vi "Test Read Arrays.vi"(11 "TwinCAT ADS in":refnum<class "TwinCAT ADS.lvclass">) -> (3 "TwinCAT ADS out":refnum<class "TwinCAT ADS.lvclass">)   [LabVIEW 2018]
uses:
  TwinCAT ADS Class/TwinCAT ADS.lvclass
  Controls/ST_Complex.ctl
  Controls/Enum.ctl
  Controls/ST_Simple.ctl
  Controls/ST_Packed.ctl
  Controls/FB_Simple.ctl
  Controls/FB_Complex.ctl
  Controls/FB_Packed.ctl
  efa47bad-600a-438a-a84b-18a2d0bd5ed2.vi
  ee10bb5d-8528-4d89-b762-575e451c5044.vi
  55aabb0d-44ac-4cb0-b0b9-4848951ad384.vi
  322127f1-f009-44a9-8110-edacd942befb.vi
  88bbdbaa-0963-4497-b00e-77a7b5e38a5d.vi
  93c90ac2-55b6-4b22-b505-e684b3e479fa.vi
  1b7d90d0-fd5f-4b83-bacb-e5e8491709de.vi
  0e82c4fa-873b-4361-ac99-2e6e4b7cd392.vi
  da0f88be-82f8-4e5b-86e7-5baa69d9b51e.vi
  4782b519-43e7-4b8e-bd72-e209be860882.vi
  e7a7b24b-aede-49d7-b369-bb451e1de87e.vi
  TwinCAT ADS Class/VIs/Data/Read.vi
  <vilib>/addons/_JKI Toolkits/Caraya/classes/Assert/Assert Equal Value and Type_Variant.vi
  <vilib>/addons/_JKI Toolkits/Caraya/classes/Assert/Assert True.vi
  <vilib>/addons/_JKI Toolkits/Caraya/classes/Assert/Assert.lvclass
  <vilib>/addons/_JKI Toolkits/Caraya/classes/Test/Test.lvclass
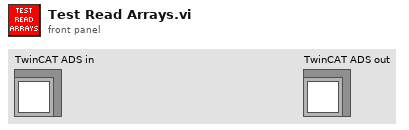
[diagram p1: front panel]
types:
  T1 = typedef "FB_Complex.ctl" = cluster{"_fMember":dbl, "_stMember":T2, "_fbSimpleMember":T6, "_fbPackedMember":T7}
  T2 = typedef "ST_Complex.ctl" = cluster{"bMember":bool, "eMember":T3, "stSimpleMember":T4, "stPackedMember":T5, "FB_Simple":T6, "arrfMember":dbl[]}
  T3 = typedef "Enum.ctl" = enum16{"Member 0", "Member 1", "Member 2"}
  T4 = typedef "ST_Simple.ctl" = cluster{"bMember":bool, "dtMember":timestamp, "nMember":i32}
  T5 = typedef "ST_Packed.ctl" = cluster{"bMember":bool, "dtMember":timestamp, "fMember":dbl}
  T6 = typedef "FB_Simple.ctl" = cluster{"_bMember":bool, "_nMember":i32, "_sMember":string}
  T7 = typedef "FB_Packed.ctl" = cluster{"bMember":bool, "nMember":i32, "sMember":string}
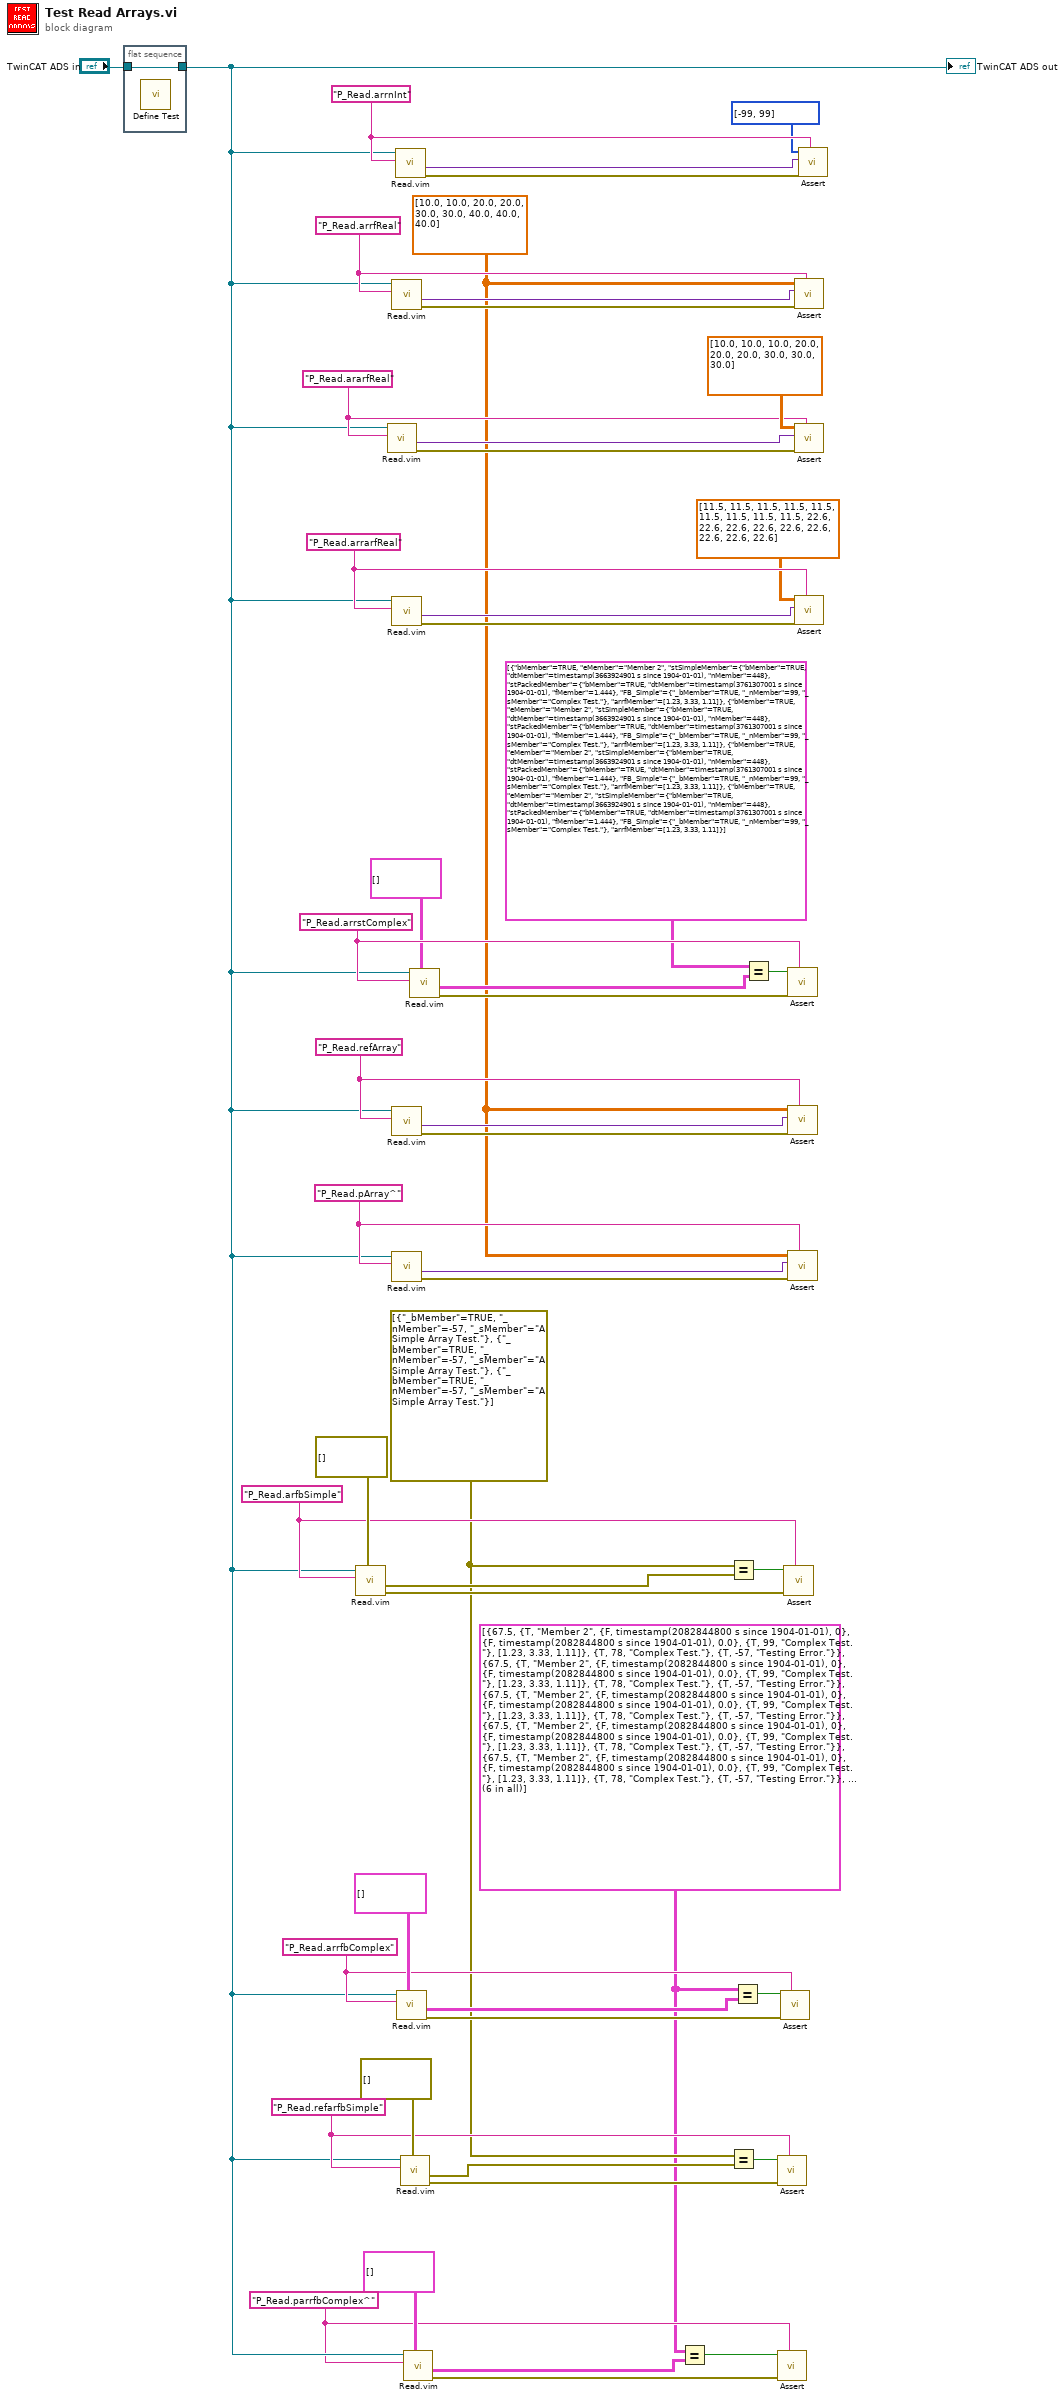
[diagram p0: block diagram]
diagram:
  w4 = "P_Read.parrfbComplex^" ("Symbol Name")
  w9 = "P_Read.refarfbSimple" ("Symbol Name")
  w15 = "P_Read.arrfbComplex" ("Symbol Name")
  w1 = T1[][] [[{"_fMember"=67.5, "_stMember"={"bMember"=TRUE, "eMember"=enum."Member 2", "stSimpleMember"={"bMember"=FALSE, "dtMember"=timestamp(2082844800 s since 1904-01-01), "nMember"=0}, "stPackedMember"={"bMember"=FALSE, "dtMember"=timestamp(2082844800 s since 1904-01-01), "fMember"=0.0}, "FB_Simple"={"_bMember"=TRUE, "_nMember"=99, "_sMember"="Complex Test."}, "arrfMember"=[1.23, 3.33, 1.11]}, "_fbSimpleMember"={"_bMember"=TRUE, "_nMember"=78, "_sMember"="Complex Test."}, "_fbPackedMember"={"bMember"=TRUE, "nMember"=-57, "sMember"="Testing Error."}}, {"_fMember"=67.5, "_stMember"={"bMember"=TRUE, "eMember"=enum."Member 2", "stSimpleMember"={"bMember"=FALSE, "dtMember"=timestamp(2082844800 s since 1904-01-01), "nMember"=0}, "stPackedMember"={"bMember"=FALSE, "dtMember"=timestamp(2082844800 s since 1904-01-01), "fMember"=0.0}, "FB_Simple"={"_bMember"=TRUE, "_nMember"=99, "_sMember"="Complex Test."}, "arrfMember"=[1.23, 3.33, 1.11]}, "_fbSimpleMember"={"_bMember"=TRUE, "_nMember"=78, "_sMember"="Complex Test."}, "_fbPackedMember"={"bMember"=TRUE, "nMember"=-57, "sMember"="Testing Error."}}], [{"_fMember"=67.5, "_stMember"={"bMember"=TRUE, "eMember"=enum."Member 2", "stSimpleMember"={"bMember"=FALSE, "dtMember"=timestamp(2082844800 s since 1904-01-01), "nMember"=0}, "stPackedMember"={"bMember"=FALSE, "dtMember"=timestamp(2082844800 s since 1904-01-01), "fMember"=0.0}, "FB_Simple"={"_bMember"=TRUE, "_nMember"=99, "_sMember"="Complex Test."}, "arrfMember"=[1.23, 3.33, 1.11]}, "_fbSimpleMember"={"_bMember"=TRUE, "_nMember"=78, "_sMember"="Complex Test."}, "_fbPackedMember"={"bMember"=TRUE, "nMember"=-57, "sMember"="Testing Error."}}, {"_fMember"=67.5, "_stMember"={"bMember"=TRUE, "eMember"=enum."Member 2", "stSimpleMember"={"bMember"=FALSE, "dtMember"=timestamp(2082844800 s since 1904-01-01), "nMember"=0}, "stPackedMember"={"bMember"=FALSE, "dtMember"=timestamp(2082844800 s since 1904-01-01), "fMember"=0.0}, "FB_Simple"={"_bMember"=TRUE, "_nMember"=99, "_sMember"="Complex Test."}, "arrfMember"=[1.23, 3.33, 1.11]}, "_fbSimpleMember"={"_bMember"=TRUE, "_nMember"=78, "_sMember"="Complex Test."}, "_fbPackedMember"={"bMember"=TRUE, "nMember"=-57, "sMember"="Testing Error."}}], [{"_fMember"=67.5, "_stMember"={"bMember"=TRUE, "eMember"=enum."Member 2", "stSimpleMember"={"bMember"=FALSE, "dtMember"=timestamp(2082844800 s since 1904-01-01), "nMember"=0}, "stPackedMember"={"bMember"=FALSE, "dtMember"=timestamp(2082844800 s since 1904-01-01), "fMember"=0.0}, "FB_Simple"={"_bMember"=TRUE, "_nMember"=99, "_sMember"="Complex Test."}, "arrfMember"=[1.23, 3.33, 1.11]}, "_fbSimpleMember"={"_bMember"=TRUE, "_nMember"=78, "_sMember"="Complex Test."}, "_fbPackedMember"={"bMember"=TRUE, "nMember"=-57, "sMember"="Testing Error."}}, {"_fMember"=67.5, "_stMember"={"bMember"=TRUE, "eMember"=enum."Member 2", "stSimpleMember"={"bMember"=FALSE, "dtMember"=timestamp(2082844800 s since 1904-01-01), "nMember"=0}, "stPackedMember"={"bMember"=FALSE, "dtMember"=timestamp(2082844800 s since 1904-01-01), "fMember"=0.0}, "FB_Simple"={"_bMember"=TRUE, "_nMember"=99, "_sMember"="Complex Test."}, "arrfMember"=[1.23, 3.33, 1.11]}, "_fbSimpleMember"={"_bMember"=TRUE, "_nMember"=78, "_sMember"="Complex Test."}, "_fbPackedMember"={"bMember"=TRUE, "nMember"=-57, "sMember"="Testing Error."}}]]
  w20 = "P_Read.arfbSimple" ("Symbol Name")
  w2 = T6[] [{"_bMember"=TRUE, "_nMember"=-57, "_sMember"="A Simple Array Test."}, {"_bMember"=TRUE, "_nMember"=-57, "_sMember"="A Simple Array Test."}, {"_bMember"=TRUE, "_nMember"=-57, "_sMember"="A Simple Array Test."}]
  w26 = "P_Read.pArray^" ("Symbol Name")
  w35 = "P_Read.arrarfReal" ("Symbol Name")
  w37 = "P_Read.ararfReal" ("Symbol Name")
  w25 = sgl[][] [[10.0, 10.0, 20.0], [20.0, 30.0, 30.0], [40.0, 40.0, 40.0]]
  w47 = "P_Read.refArray" ("Symbol Name")
  w48 = "P_Read.arrstComplex" ("Symbol Name")
  w43 = "P_Read.arrfReal" ("Symbol Name")
  w50 = "P_Read.arrnInt" ("Symbol Name")
  n1 = flat-sequence {
    tunnel: "TwinCAT ADS in" -> [w53]
    tunnel: [w53] -> w7
    frame #0 {
      n2 = call <vilib>:"Define Test.vi"() -> ()  [unwired: 10 in, 2 out]
    }
  }
  n3 = call "Read.vim"("Type"=T6[] [], "Symbol Name"=w20, "TwinCAT ADS in"=w7) -> ("error out"=w22:errorcluster, "Value"=w10:T6[])  [unwired: 6 in, 1 out]
  n4 = call "Read.vim"("Symbol Name"=w37, "TwinCAT ADS in"=w7) -> ("error out"=w40:errorcluster, "Value"=w39:variant)  [unwired: 7 in, 1 out]
  n5 = call "Read.vim"("Symbol Name"=w43, "TwinCAT ADS in"=w7) -> ("error out"=w49:errorcluster, "Value"=w41:variant)  [unwired: 7 in, 1 out]
  n6 = call "Read.vim"("Symbol Name"=w35, "TwinCAT ADS in"=w7) -> ("error out"=w36:errorcluster, "Value"=w33:variant)  [unwired: 7 in, 1 out]
  n7 = call "Read.vim"("Symbol Name"=w47, "TwinCAT ADS in"=w7) -> ("error out"=w46:errorcluster, "Value"=w32:variant)  [unwired: 7 in, 1 out]
  n8 = call "Read.vim"("Symbol Name"=w26, "TwinCAT ADS in"=w7) -> ("error out"=w27:errorcluster, "Value"=w24:variant)  [unwired: 7 in, 1 out]
  n9 = call "Read.vim"("Symbol Name"=w50, "TwinCAT ADS in"=w7) -> ("error out"=w52:errorcluster, "Value"=w45:variant)  [unwired: 7 in, 1 out]
  n10 = call "Read.vim"("Type"=T1[][] [], "Symbol Name"=w15, "TwinCAT ADS in"=w7) -> ("error out"=w19:errorcluster, "Value"=w18:T1[][])  [unwired: 6 in, 1 out]
  n11 = call "Read.vim"("Type"=T6[] [], "Symbol Name"=w9, "TwinCAT ADS in"=w7) -> ("error out"=w12:errorcluster, "Value"=w11:T6[])  [unwired: 6 in, 1 out]
  n12 = call "Read.vim"("Type"=T1[][] [], "Symbol Name"=w4, "TwinCAT ADS in"=w7) -> ("error out"=w6:errorcluster, "Value"=w3:T1[][])  [unwired: 6 in, 1 out]
  n13 = call "Read.vim"("Type"=T2[][] [], "Symbol Name"=w48, "TwinCAT ADS in"=w7) -> ("error out"=w42:errorcluster, "Value"=w29:T2[][])  [unwired: 6 in, 1 out]
  n14 = Equal?(x=w1, y=w3) -> (x = y?=w5:bool)
  n15 = Equal?(x=w2, y=w10) -> (x = y?=w21:bool)
  n16 = Equal?(x=w2, y=w11) -> (x = y?=w13:bool)
  n17 = Equal?(x=w1, y=w18) -> (x = y?=w17:bool)
  n18 = Equal?(x=T2[][] [[{"bMember"=TRUE, "eMember"=enum."Member 2", "stSimpleMember"={"bMember"=TRUE, "dtMember"=timestamp(3663924901 s since 1904-01-01), "nMember"=448}, "stPackedMember"={"bMember"=TRUE, "dtMember"=timestamp(3761307001 s since 1904-01-01), "fMember"=1.444}, "FB_Simple"={"_bMember"=TRUE, "_nMember"=99, "_sMember"="Complex Test."}, "arrfMember"=[1.23, 3.33, 1.11]}, {"bMember"=TRUE, "eMember"=enum."Member 2", "stSimpleMember"={"bMember"=TRUE, "dtMember"=timestamp(3663924901 s since 1904-01-01), "nMember"=448}, "stPackedMember"={"bMember"=TRUE, "dtMember"=timestamp(3761307001 s since 1904-01-01), "fMember"=1.444}, "FB_Simple"={"_bMember"=TRUE, "_nMember"=99, "_sMember"="Complex Test."}, "arrfMember"=[1.23, 3.33, 1.11]}], [{"bMember"=TRUE, "eMember"=enum."Member 2", "stSimpleMember"={"bMember"=TRUE, "dtMember"=timestamp(3663924901 s since 1904-01-01), "nMember"=448}, "stPackedMember"={"bMember"=TRUE, "dtMember"=timestamp(3761307001 s since 1904-01-01), "fMember"=1.444}, "FB_Simple"={"_bMember"=TRUE, "_nMember"=99, "_sMember"="Complex Test."}, "arrfMember"=[1.23, 3.33, 1.11]}, {"bMember"=TRUE, "eMember"=enum."Member 2", "stSimpleMember"={"bMember"=TRUE, "dtMember"=timestamp(3663924901 s since 1904-01-01), "nMember"=448}, "stPackedMember"={"bMember"=TRUE, "dtMember"=timestamp(3761307001 s since 1904-01-01), "fMember"=1.444}, "FB_Simple"={"_bMember"=TRUE, "_nMember"=99, "_sMember"="Complex Test."}, "arrfMember"=[1.23, 3.33, 1.11]}]], y=w29) -> (x = y?=w31:bool)
  n19 = call-poly <vilib>:"Assert.vi"("Label"=w9, "error in (no error)"=w12, "True?"=w13) -> ()  [unwired: 7 in, 2 out]
  n20 = call-poly <vilib>:"Assert.vi"("Label"=w4, "error in (no error)"=w6, "True?"=w5) -> ()  [unwired: 7 in, 2 out]
  n21 = call-poly <vilib>:"Assert.vi"("Label"=w15, "error in (no error)"=w19, "True?"=w17) -> ()  [unwired: 7 in, 2 out]
  n22 = call-poly <vilib>:"Assert.vi"("Label"=w20, "error in (no error)"=w22, "True?"=w21) -> ()  [unwired: 7 in, 2 out]
  n23 = call-poly <vilib>:"Assert.vi"("Label"=w48, "error in (no error)"=w42, "True?"=w31) -> ()  [unwired: 7 in, 2 out]
  n24 = call-poly <vilib>:"Assert.vi"("Label"=w47, "error in (no error)"=w46, "Y"=w32, "X"=w25) -> ()  [unwired: 6 in, 2 out]
  n25 = call-poly <vilib>:"Assert.vi"("Label"=w26, "error in (no error)"=w27, "Y"=w24, "X"=w25) -> ()  [unwired: 6 in, 2 out]
  n26 = call-poly <vilib>:"Assert.vi"("Label"=w43, "error in (no error)"=w49, "Y"=w41, "X"=w25) -> ()  [unwired: 6 in, 2 out]
  n27 = call-poly <vilib>:"Assert.vi"("Label"=w37, "error in (no error)"=w40, "Y"=w39, "X"=sgl[][] [[10.0, 10.0, 10.0], [20.0, 20.0, 20.0], [30.0, 30.0, 30.0]]) -> ()  [unwired: 6 in, 2 out]
  n28 = call-poly <vilib>:"Assert.vi"("Label"=w35, "error in (no error)"=w36, "Y"=w33, "X"=dbl[][][] [[[11.5, 11.5, 11.5], [11.5, 11.5, 11.5], [11.5, 11.5, 11.5]], [[22.6, 22.6, 22.6], [22.6, 22.6, 22.6], [22.6, 22.6, 22.6]]]) -> ()  [unwired: 6 in, 2 out]
  n29 = call-poly <vilib>:"Assert.vi"("Label"=w50, "error in (no error)"=w52, "Y"=w45, "X"=i16[] [-99, 99]) -> ()  [unwired: 6 in, 2 out]
  "TwinCAT ADS out" <- w7
